vi "Test connection.vi"(11 "Connection Type":string) -> (0 "error out":errorcluster, 3 "Error string":string)   [LabVIEW 2018]
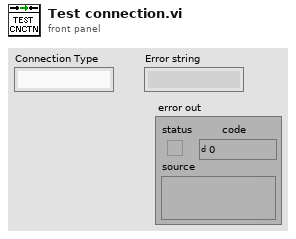
[diagram p1: front panel]
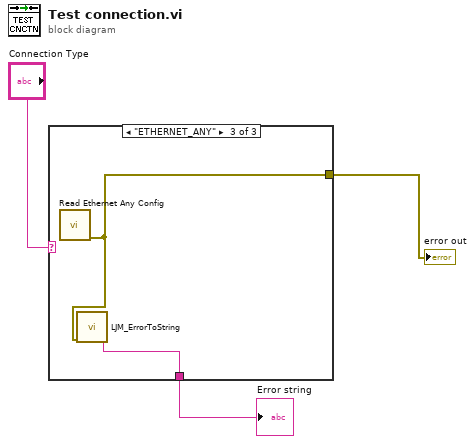
[diagram p0: block diagram]
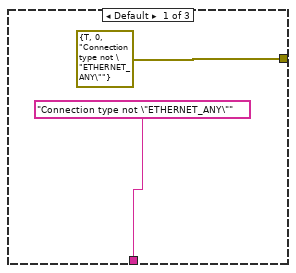
[diagram p2: hidden frame]
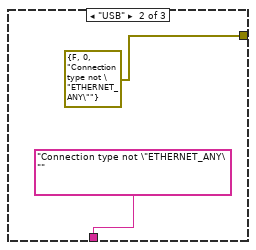
[diagram p3: hidden frame]
diagram:
  n1 = case shown="\"ETHERNET_ANY\"" "Connection Type" {
    tunnel: ["Connection type not \"ETHERNET_ANY\"" "Connection type not \"ETHERNET_ANY\"" ("source") w9] -> w3
    tunnel: [errorcluster {"status"=TRUE, "code"=0, "source"="Connection type not \"ETHERNET_ANY\""} ("error constant") errorcluster {"status"=FALSE, "code"=0, "source"="Connection type not \"ETHERNET_ANY\""} ("error constant") w8] -> w1
    frame Default {
    }
    frame "USB" {
    }
    frame "ETHERNET_ANY" {
      n2 = call "Read Ethernet Any Config.vi"() -> ("error out"=w8:errorcluster)  [unwired: 11 in]
      n3 = call "LJM_ErrorToString.vi"("error in"=w8) -> ("String"=w9:string)  [unwired: 10 in]
    }
  }
  "Error string" <- w3
  "error out" <- w1
